vi "GetScaling.vi"(8 "error in (no error)":errorcluster, 11 "Subsystem":refnum<class "DAQmx(AI).lvclass">) -> (0 "error out":errorcluster, 1 "Custom Scaling":bool, 2 "Scaling":T1={"Scale Name"="SMO-Sim/ai0", "Scale Type"=enum."Map Range", "Scaled Units"="SMO-Sim/ai0", "Linear"={"Slope"=1.0, "Intercept"=0.0}, "Map Range"={"Minimum"=1.0, "Maximum"=0.0}, "Polynomial"={"forward coeff"=[], "reverse coeff"=[]}, "Table"={"scaled values"=[], "pres-scaled values"=[]}}, 3 "Subsystem out":refnum<class "DAQmx(AI).lvclass">)   [LabVIEW 2019, in "DAQmx(AI).lvclass"]
doc: "---------------------------------------------------------------\nJKI State Machine Objects™\nhttp://jki.net/state-machine-objects/\nCopyright (C) 2005-2015, JKI <info@jki.net>\nALL RIGHTS RESERVEDJKI State Machine Objects (SMO) 1.0.0.5\nJKI - JKI\nCopyright (c) 2016, JKI"
uses:
  DAQmx(AI).lvclass
  Typedefs/Scaling--Cluster.ctl
  Typedefs/ScalingType--Enum.ctl
  Typedefs/Scaling(Linear)--Cluster.ctl
  Typedefs/Scaling(MapRange)--Cluster.ctl
  Typedefs/Scaling(Polynomial)--Cluster.ctl
  Typedefs/Scaling(Table)--Cluster.ctl
  DAQmx(AI).lvclass/DAQmx(AI).ctl
panel:
  # "For instructions on how to use the JKI State Machine Objects, examples and video tutorials, visit:\nhttp://jki.net/state-machine-objects/\n\nJKI State Machine Objects™\nhttp://jki.net/state-machine-objects/\nCopyright (C) 2005-2015, JKI <info@jki.net>\nALL RIGHTS RESERVED"
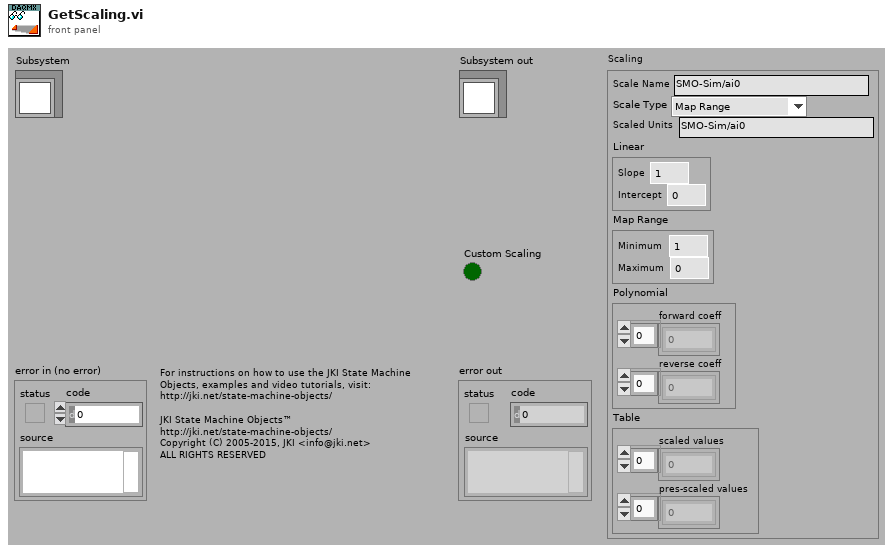
[diagram p1: front panel]
types:
  T1 = typedef "DAQmx(AI).lvclass/Scaling--Cluster.ctl" = cluster{"Scale Name":string, "Scale Type":T2, "Scaled Units":string, "Linear":T3, "Map Range":T4, "Polynomial":T5, "Table":T6}
  T2 = typedef "DAQmx(AI).lvclass/ScalingType--Enum.ctl" = enum16{"No scaling", "Linear", "Map Range", "Polynomial", "Table"}
  T3 = typedef "DAQmx(AI).lvclass/Scaling(Linear)--Cluster.ctl" = cluster{"Slope":dbl, "Intercept":dbl}
  T4 = typedef "DAQmx(AI).lvclass/Scaling(MapRange)--Cluster.ctl" = cluster{"Minimum":dbl, "Maximum":dbl}
  T5 = typedef "DAQmx(AI).lvclass/Scaling(Polynomial)--Cluster.ctl" = cluster{"forward coeff":dbl[], "reverse coeff":dbl[]}
  T6 = typedef "DAQmx(AI).lvclass/Scaling(Table)--Cluster.ctl" = cluster{"scaled values":dbl[], "pres-scaled values":dbl[]}
  T7 = typedef "DAQmx(AI).lvclass/PrivateData--Ref.ctl" = refnum<data-value>
  T8 = typedef "DAQmx(AI).lvclass/PrivateData--Cluster.ctl" = cluster{"Configuration":T9, "Public Events":T11, "Data":dbl, "Scaling":T1, "Private Events":T12}
  T9 = typedef "DAQmx(AI).lvclass/Configuration--Cluster.ctl" = cluster{"PhysChan":tag, "Period (ms)":i64, "input terminal cfg":i32, "minimum value":dbl, "maximum value":dbl, "units":T10, "task name":string, "TDMS File Path":path, "Group Name":string}
  T10 = typedef "DAQmx(AI).lvclass/Units -- Enum.ctl" = enum16{"Volts", "Amps", "Deg F", "Deg C", "Deg R", "Kelvins", "Strain", "Ohms", "Hz", "Seconds", "Meters", "Inches", "Degrees", "Radians", "Ticks", "g", "m/s^2", "m/s", "in/s", "Pascals", "Newtons", "Pounds", "kgf", "psi", "bar", "Nm", "oz-in", "lb-in", "lb-ft", "Volts/Volt", "mVolts/Volt", "From TEDS"}
  T11 = typedef "DAQmx(AI).lvclass/PublicEvents--Cluster.ctl" = cluster{"Value Changed":refnum<user-event>, "Task Configuration":refnum<user-event>, "Scaling":refnum<user-event>}
  T12 = typedef "DAQmx(AI).lvclass/PrivateEvents--Cluster.ctl" = cluster{"Logging":refnum<user-event>}
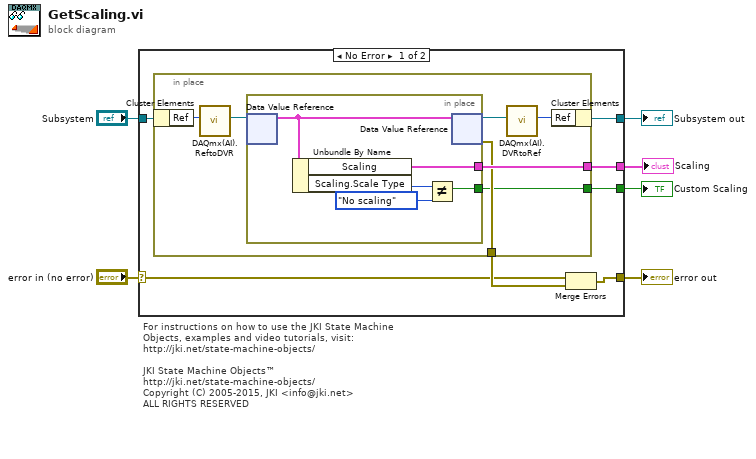
[diagram p0: block diagram]
diagram:
  # "For instructions on how to use the JKI State Machine Objects, examples and video tutorials, visit:\nhttp://jki.net/state-machine-objects/\n\nJKI State Machine Objects™\nhttp://jki.net/state-machine-objects/\nCopyright (C) 2005-2015, JKI <info@jki.net>\nALL RIGHTS RESERVED"
  n1 = case shown="No Error" "error in (no error)" {
    selector: "error in (no error)" -> [w8 w26]
    tunnel: "Subsystem" -> [w9 w27]
    tunnel: [w10 w26] -> w5
    tunnel: [w13 w27] -> w4
    tunnel: [w12 _] -> w2
    tunnel: [w7 _] -> w1
    frame No Error {
      n2 = in-place {
        in-place-border: [w20] -> w12
        in-place-border: [w19] -> w11
        in-place-border: [w14] -> w7
        n3 = in-place-cluster #1(w9) -> ("Ref"=w18:u32)
        n4 = call "DAQmx(AI).ReftoDVR.vi"("Ref"=w18) -> ("Ref"=w17:T7)  [unwired: 10 in]
        n5 = in-place {
          in-place-border: [w24] -> w20
          in-place-border: [w21] -> w14
          n6 = in-place-dvr #2(w17) -> (w25:T8)  [unwired: 1 out]
          n7 = Unbundle By Name(w25) -> ("Scaling"=w24:T1, "Scaling.Scale Type"=w23:T2)
          n8 = Not Equal?(x=w23, y=ScalingType--Enum."No scaling") -> (x != y?=w21:bool)
          n9 = in-place-dvr #2(w25) -> (w16:T7, w19:errorcluster)
        }
        n10 = call "DAQmx(AI).DVRtoRef.vi"("Ref"=w16) -> ("Ref"=w15:u32)  [unwired: 10 in]
        n11 = in-place-cluster #1("Ref"=w15) -> (w13:refnum<class "DAQmx(AI).lvclass">)
      }
      n12 = Merge Errors(w8, w11) -> (w10:errorcluster)
    }
    frame Error {
    }
  }
  "error out" <- w5
  "Subsystem out" <- w4
  "Scaling" <- w2
  "Custom Scaling" <- w1
